vi "Test Dynamic Failing Method.vi"(8 "error in (no error)":errorcluster, 11 "Test Case Skipping Inherited Method in":refnum<class "Test Case Skipping Inherited Method.lvclass">) -> (0 "error out":errorcluster, 3 "Test Case Skipping Inherited Method out":refnum<class "Test Case Skipping Inherited Method.lvclass">)   [LabVIEW 2020, in "Test Case Skipping Inherited Method.lvclass"]
uses:
  Test Case Skipping Inherited Method.lvclass
  C:/Git/astemes-lunit/source/Framework/Test Case/LUnit Test Case.lvclass
  source/Framework/Test Case/LUnit Test Case.lvclass/LUnit Test Case.ctl
  source/Framework/Test Case/Private/SubVIs/Add test result.vi
  source/Framework/Test Case/Private/SubVIs/Set Assertion Type.vi
  source/Framework/Result Types/Case Result/Public/Record Assertion Result.vi
  source/Framework/Result Types/Method Result/Public/Aggregate Assertion Results.vi
  source/Framework/Result Types/Method Result/Private/Merge Status.vi
  source/Framework/Result Types/Method Result/Private/Concatenate result strings.vi
  source/Framework/Test Case/LUnit Test Case.lvclass
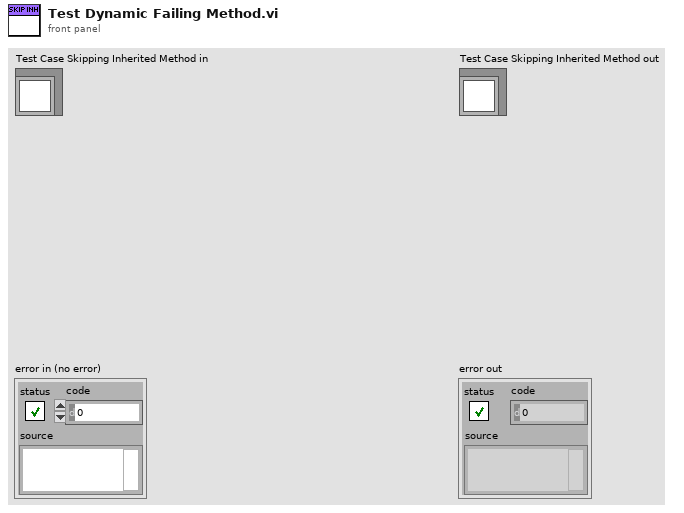
[diagram p1: front panel]
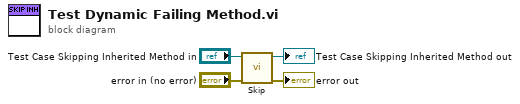
[diagram p0: block diagram]
diagram:
  n1 = call "Skip.vi"("error in (no error)"="error in (no error)", "LUnit Test Case In"="Test Case Skipping Inherited Method in") -> ("error out"=→"error out":errorcluster, "LUnit Test Case Out"=→"Test Case Skipping Inherited Method out":refnum<class "Test Case Skipping Inherited Method.lvclass">)  [unwired: 8 in]
